vi "Condition Rewire From Bundle.vi"(6 "IO":T1, 8 "error in":errorcluster, 9 "Name":string, 10 "VI?":refnum<vi>) -> (0 "error out":errorcluster)   [LabVIEW 2020, in "_Rescript.lvlib" / "Msg.lvlib" / "Msg.lvclass"]
uses:
  Msg.lvclass
  IO.ctl
  <vilib>/Utility/traverseref.llb/TRef TravTarget.ctl
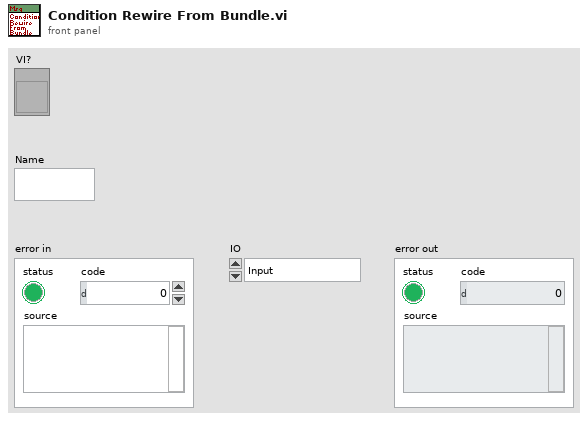
[diagram p1: front panel]
types:
  T1 = typedef "_Rescript.lvlib/Msg.lvlib/Msg.lvclass/IO.ctl" = enum16{"Input", "Output"}
  T2 = typedef "TRef TravTarget.ctl" = enum16{"FP", "BD", "Other"}
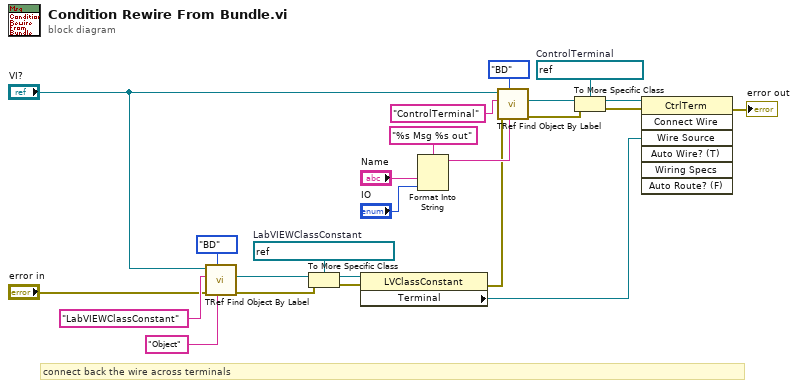
[diagram p0: block diagram]
diagram:
  w10 = refnum<vi> refnum  # ControlTerminal
  w22 = refnum<vi> refnum  # LabVIEWClassConstant
  # "connect back the wire across terminals"
  n1 = call <vilib>:"TRef Find Object By Label.vi"("Label"="Object", "Traverse Target"=TRef_TravTarget."BD", "error in (no error)"="error in", "Class Name"="LabVIEWClassConstant", "VI Ref"="VI?") -> ("error out"=w23:errorcluster, "Found Obj Ref"=w21:refnum<vi>)  [unwired: 3 in, 2 out]
  n2 = To More Specific Class(target class=w22, reference=w21, error in=w23) -> (specific class reference=w18:refnum<vi>, error out=w16:errorcluster)
  n3 = property class="LVClassConstant"(reference=w18, error in=w16) -> (error out=w7:errorcluster, "Terminal"=w5:refnum<vi>)  [unwired: 1 out]
  n4 = Format Into String(format string="%s Msg %s out", "Name", "IO") -> (resulting string=w13:string)  [unwired: 2 in, 1 out]
  n5 = call <vilib>:"TRef Find Object By Label.vi"("Label"=w13, "Traverse Target"=TRef_TravTarget."BD", "error in (no error)"=w7, "Class Name"="ControlTerminal", "VI Ref"="VI?") -> ("error out"=w11:errorcluster, "Found Obj Ref"=w12:refnum<vi>)  [unwired: 3 in, 2 out]
  n6 = To More Specific Class(target class=w10, reference=w12, error in=w11) -> (specific class reference=w8:refnum<vi>, error out=w6:errorcluster)
  n7 = invoke class="CtrlTerm" method="Connect Wire"(reference=w8, error in=w6, "Wire Source"=w5) -> (error out=→"error out":errorcluster)  [unwired: 4 in, 6 out]
